vi "TCPDeviceNameRead.vi"(8 "error in (no error)":errorcluster, 11 "connection ID":refnum<k5>) -> (0 "error out":errorcluster, 1 "empty?":bool, 2 "TCPDeviceName":string, 3 "connection ID out":refnum<k5>)   [LabVIEW 2020]
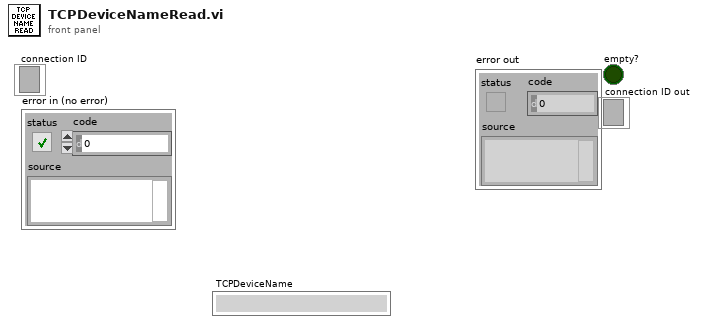
[diagram p1: front panel]
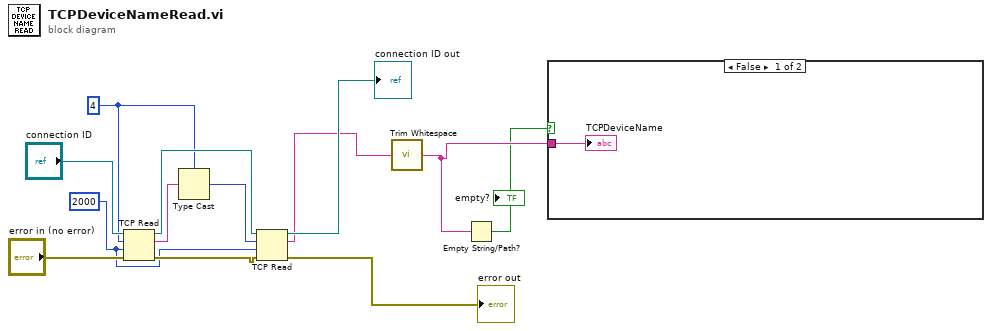
[diagram p0: block diagram]
diagram:
  w9 = 4
  w1 = 2000 ("timeout ms (25000)")
  n1 = TCP Read(connection ID="connection ID", bytes to read=w9, error in (no error)="error in (no error)", 9:w1) -> (connection ID out=w13:refnum<k5>, data out=w12:string, error out=w3:errorcluster)  [unwired: 1 in]
  n2 = Type Cast(type=w9, x=w12) -> (*(type *) &x=w8:i32)
  n3 = TCP Read(connection ID=w13, bytes to read=w8, error in (no error)=w3, 9:w1) -> (connection ID out=→"connection ID out":refnum<k5>, data out=w5:string, error out=→"error out":errorcluster)  [unwired: 1 in]
  n4 = call <vilib>:"Trim Whitespace.vi"("string"=w5) -> ("trimmed string"=w4:string)  [unwired: 1 in]
  n5 = Empty String/Path?(string/path=w4) -> (empty?=w2:bool)
  "empty?" <- w2
  n6 = case shown="False" w2 {
    tunnel: w4 -> [w14 _]
    frame False {
      "TCPDeviceName" <- w14
    }
    frame True {
    }
  }
